vi "Module Loop.vi"(8 "error in (no error)":errorcluster, 11 "PluginGUI in":refnum<class "PluginGUI.lvclass">) -> (0 "error out":errorcluster, 3 "PluginGUI out":refnum<class "PluginGUI.lvclass">)   [LabVIEW 2020, in "VolatusGUI.lvlib" / "PluginGUI.lvclass"]
uses:
  PluginGUI.lvclass
  C:/dev/lv20CE/relink/lv-volatus/Volatus/Module/Module.lvclass
  Volatus/Module/Module.lvclass
  PluginGUI.lvclass/PluginGUI.ctl
  GUI Info.ctl
  Volatus/Show GUI Options.ctl
  Volatus/Module/Module.lvclass/Module.ctl
  <vilib>/Utility/error.llb/Error Cluster From Error Code.vi
  GUI Helper/GUI Helper.lvclass
  Volatus/Volatus.lvlib
  VolatusGUI.lvlib
  C:/dev/lv20CE/relink/lv-volatus/VolatusGUI/PluginGUI/PluginGUI.lvclass
  Volatus/Roles API/Roles API.lvclass
panel:
  out "VI Name":string
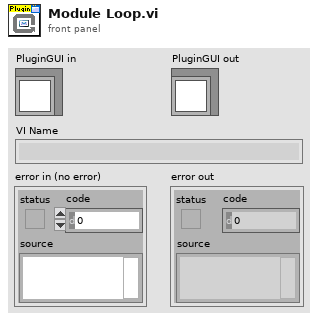
[diagram p1: front panel]
types:
  T1 = typedef "VolatusGUI.lvlib/GUI Info.ctl" = cluster{"Color":u32, "Name":string}
  T2 = typedef "Volatus.lvlib/Show GUI Options.ctl" = cluster{"Show Core Module":bool}
  T3 = enum32{"Invalid", "Standard", "Closed", "Hidden", "Minimized", "Maximized"}
  T4 = typedef "VolatusGUI.lvlib/PluginGUI.lvclass/GUI Type.ctl" = enum16{"Unknown", "Config", "Path", "Ref"}
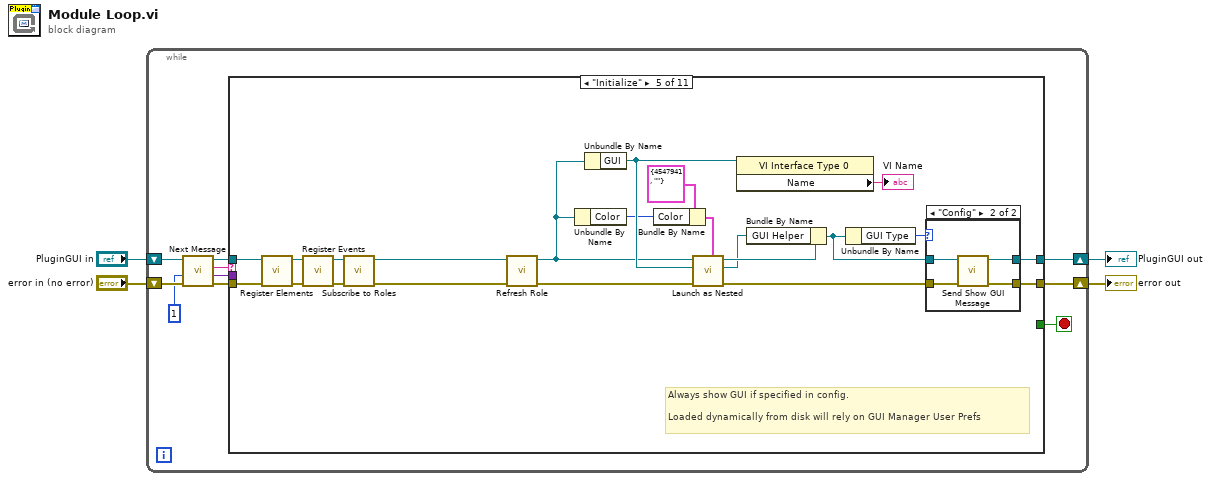
[diagram p0: block diagram]
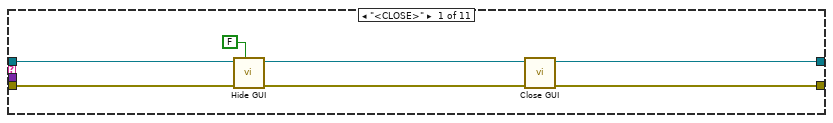
[diagram p2: hidden frame]
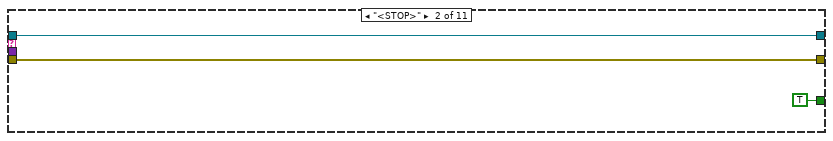
[diagram p3: hidden frame]
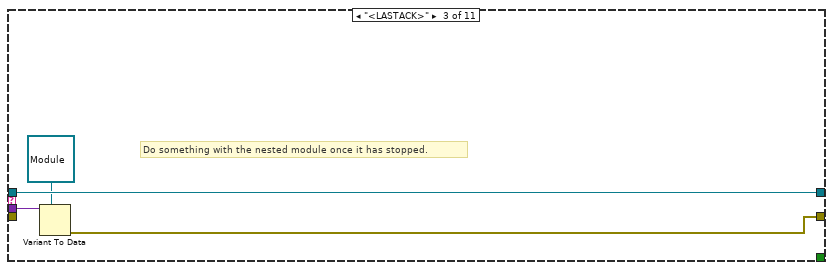
[diagram p4: hidden frame]
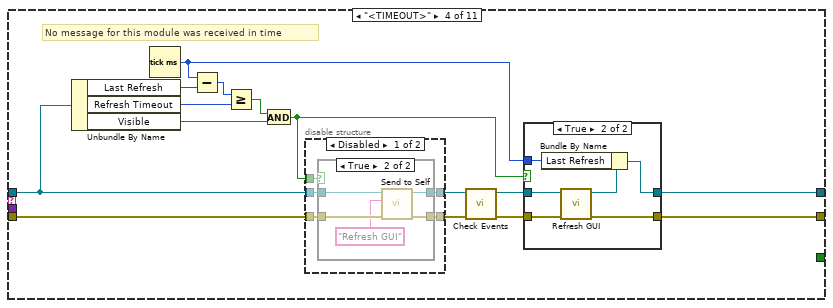
[diagram p5: hidden frame]
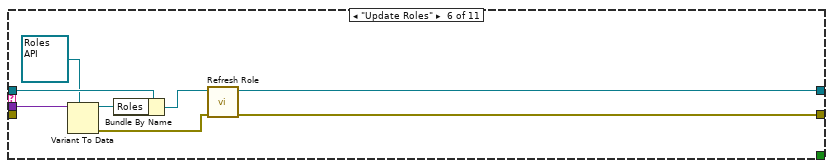
[diagram p10: hidden frame]
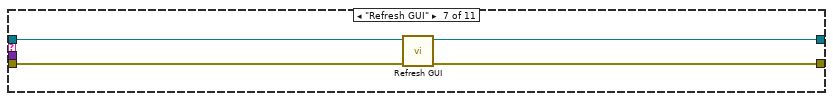
[diagram p11: hidden frame]
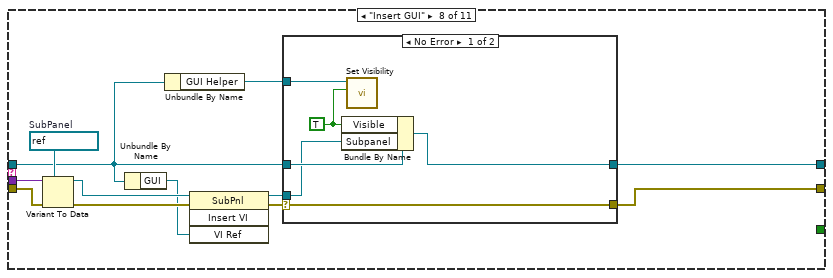
[diagram p12: hidden frame]
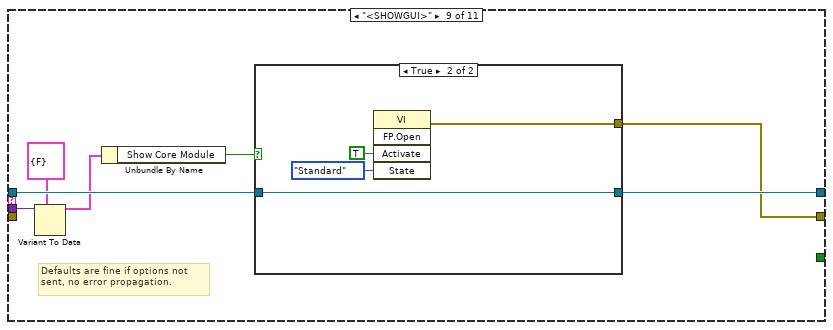
[diagram p14: hidden frame]
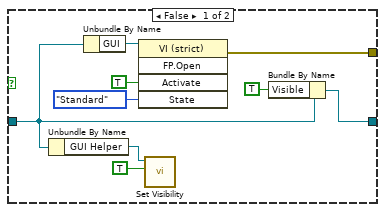
[diagram p15: hidden frame]
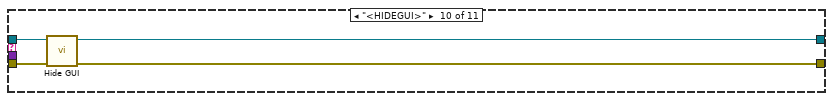
[diagram p16: hidden frame]
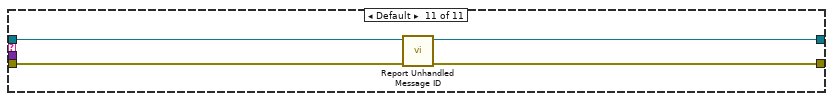
[diagram p17: hidden frame]
diagram:
  n1 = while {
    shift-right: [w9] -> w3
    shift-left: "PluginGUI in" -> [w14]
    shift-right: [w8] -> w2
    shift-left: "error in (no error)" -> [w13]
    stop <- w7 stop-if-true
    n2 = call "Next Message.vi"("error in (no error)"=w13, "Timeout ms (-1)"=1, "Module in"=w14) -> ("error out"=w12:errorcluster, "Data"=w6:variant, "ID"=w11:string, "Module in"=w10:refnum<class "PluginGUI.lvclass">)  [unwired: 5 in]
    n3 = case shown="\"Initialize\"" w11 {
      tunnel: w12 -> [w21 w23 _ w43 w84 _ w105 w117 _ w148 w153]
      tunnel: w10 -> [w19 w24 w28 w41 w74 w101 w103 w107 w131 w149 w151]
      tunnel: [w15 w24 w28 w31 w77 w96 w102 w109 w132 w147 w150] -> w9
      tunnel: [w17 w23 w25 w33 w78 w94 w104 w108 w126 w146 w152] -> w8
      tunnel: [_ TRUE _ _ _ _ _ _ _ _ _] -> w7
      tunnel: w6 -> [_ _ w27 _ _ w100 _ w116 w130 _ _]
      frame "<CLOSE>" {
        n4 = call "Hide GUI.vi"("Save Pref (T)"=FALSE, "error in (no error)"=w21, "PluginGUI in"=w19) -> ("error out"=w20:errorcluster, "PluginGUI out"=w16:refnum<class "PluginGUI.lvclass">)  [unwired: 7 in]
        n5 = call "Close GUI.vi"("error in (no error)"=w20, "PluginGUI in"=w16) -> ("error out"=w17:errorcluster, "PluginGUI out"=w15:refnum<class "PluginGUI.lvclass">)  [unwired: 8 in]
      }
      frame "<STOP>" {
      }
      frame "<LASTACK>" {
        # "Do something with the nested module once it has stopped."
        n6 = Variant To Data(type=refnum<class "Module.lvclass"> refnum ("Volatus:Module"), Variant=w27) -> (error out=w25:errorcluster)  [unwired: 1 in, 1 out]
      }
      frame "<TIMEOUT>" {
        # "No message for this module was received in time"
        n7 = Unbundle By Name(w41) -> ("Last Refresh"=w37:u32, "Refresh Timeout"=w36:i32, "Visible"=w40:bool)
        n8 = Tick Count (ms)() -> (millisecond timer value=w29:u32)
        n9 = Subtract(x=w29, y=w37) -> (x-y=w35:u32)
        n10 = Greater Or Equal?(x=w35, y=w36) -> (x >= y?=w34:bool)
        n11 = And(x=w34, y=w40) -> (x .and. y?=w30:bool)
        n12 = disable-structure shown="Disabled" {
          disable-tunnel: w43 -> [w56 w64]
          disable-tunnel: [w55 w64] -> w42
          disable-tunnel: w41 -> [w54 w65]
          disable-tunnel: [w53 w65] -> w38
          disable-tunnel: w30 -> [w52 _]
          frame Disabled {
            n13 = case shown="True" w52 {
              tunnel: w56 -> [w57 w63]
              tunnel: [w57 w62] -> w55
              tunnel: [w58 w61] -> w53
              tunnel: w54 -> [w58 w59]
              frame False {
              }
              frame True {
                n14 = call "Send to Self.vi"("error in (no error)"=w63, "Message ID"="Refresh GUI", "Module in"=w59) -> ("error out"=w62:errorcluster, "Module in"=w61:refnum<class "PluginGUI.lvclass">)  [unwired: 7 in]
              }
            }
          }
          frame Enabled {
          }
        }
        n15 = call "Check Events.vi"("error in (no error)"=w42, "PluginGUI in"=w38) -> ("error out"=w39:errorcluster, "PluginGUI out"=w32:refnum<class "PluginGUI.lvclass">)  [unwired: 8 in]
        n16 = case shown="True" w30 {
          tunnel: w39 -> [w44 w51]
          tunnel: [w44 w50] -> w33
          tunnel: w32 -> [w45 w49]
          tunnel: [w45 w47] -> w31
          tunnel: w29 -> [_ w46]
          frame False {
          }
          frame True {
            n17 = call "Refresh GUI.vi"("error in (no error)"=w51, "PluginGUI in"=w49) -> ("error out"=w50:errorcluster, "PluginGUI out"=w48:refnum<class "PluginGUI.lvclass">)  [unwired: 8 in]
            n18 = Bundle By Name(cluster=w48, "Last Refresh"=w46) -> (w47:refnum<class "PluginGUI.lvclass">)
          }
        }
      }
      frame "Initialize" {
        # "Always show GUI if specified in config.\n\nLoaded dynamically from disk will rely on GUI Manager User Prefs"
        n19 = call "Register Elements.vi"("error in (no error)"=w84, "PluginGUI in"=w74) -> ("error out"=w87:errorcluster, "PluginGUI out"=w85:refnum<class "PluginGUI.lvclass">)  [unwired: 8 in]
        n20 = call "Register Events.vi"("error in (no error)"=w87, "PluginGUI in"=w85) -> ("error out"=w86:errorcluster, "PluginGUI out"=w69:refnum<class "PluginGUI.lvclass">)  [unwired: 8 in]
        n21 = call "Subscribe to Roles.vi"("error in (no error)"=w86, "Module in"=w69) -> ("error out"=w70:errorcluster, "Module out"=w67:refnum<class "PluginGUI.lvclass">)  [unwired: 8 in]
        n22 = call "Refresh Role.vi"("error in (no error)"=w70, "PluginGUI in"=w67) -> ("error out"=w68:errorcluster, "PluginGUI out"=w66:refnum<class "PluginGUI.lvclass">)  [unwired: 8 in]
        n23 = Unbundle By Name(w66) -> ("Color"=w71:u32)
        n24 = Unbundle By Name(w66) -> ("GUI"=w80:refnum<vi>)
        n25 = Bundle By Name(cluster=T1 {"Color"=4547941, "Name"=""} ("GUI Info (Default)"), "Color"=w71) -> (w72:T1)
        n26 = call "Launch as Nested.vi"("GUI Info (Default)"=w72, "error in (no error)"=w68, "GUI"=w80, "Parent in"=w66) -> ("error out"=w82:errorcluster, "MessageQ"=w79:refnum<class "MessageQ.lvclass">, "Parent"=w81:refnum<class "PluginGUI.lvclass">)  [unwired: 5 in]
        n27 = property class="VI Interface Type 0"(reference=w80) -> ("Name"=→"VI Name":string)  [unwired: 1 in, 2 out]
        n28 = Bundle By Name(cluster=w81, "GUI Helper"=w79) -> (w76:refnum<class "PluginGUI.lvclass">)
        n29 = Unbundle By Name(w76) -> ("GUI Type"=w75:T4)
        n30 = case shown="\"Config\"" w75 {
          tunnel: w82 -> [w88 w93]
          tunnel: [w88 w92] -> w78
          tunnel: [w89 w91] -> w77
          tunnel: w76 -> [w89 w90]
          frame Default {
          }
          frame "Config" {
            n31 = call "Send Show GUI Message.vi"("error in (no error)"=w93, "Module in"=w90) -> ("error out"=w92:errorcluster, "Module in"=w91:refnum<class "PluginGUI.lvclass">)  [unwired: 8 in]
          }
        }
      }
      frame "Update Roles" {
        n32 = Variant To Data(type=refnum<class "Roles API.lvclass"> refnum ("Volatus:Roles API.lvclass"), Variant=w100) -> (data=w97:refnum<class "Roles API.lvclass">, error out=w95:errorcluster)  [unwired: 1 in]
        n33 = Bundle By Name(cluster=w101, "Roles"=w97) -> (w98:refnum<class "PluginGUI.lvclass">)
        n34 = call "Refresh Role.vi"("error in (no error)"=w95, "PluginGUI in"=w98) -> ("error out"=w94:errorcluster, "PluginGUI out"=w96:refnum<class "PluginGUI.lvclass">)  [unwired: 8 in]
      }
      frame "Refresh GUI" {
        n35 = call "Refresh GUI.vi"("error in (no error)"=w105, "PluginGUI in"=w103) -> ("error out"=w104:errorcluster, "PluginGUI out"=w102:refnum<class "PluginGUI.lvclass">)  [unwired: 8 in]
      }
      frame "Insert GUI" {
        w115 = refnum<vi> refnum  # SubPanel
        n36 = Variant To Data(error in=w117, type=w115, Variant=w116) -> (data=w113:refnum<vi>, error out=w114:errorcluster)
        n37 = Unbundle By Name(w107) -> ("GUI"=w112:refnum<vi>)
        n38 = Unbundle By Name(w107) -> ("GUI Helper"=w106:refnum<class "MessageQ.lvclass">)
        n39 = invoke class="SubPnl" method="Insert VI"(reference=w113, error in=w114, "VI Ref"=w112) -> (reference out=w110:refnum<vi>, error out=w111:errorcluster)  [unwired: 1 in, 2 out]
        n40 = case shown="No Error" w111 {
          selector: w111 -> [w120 w125]
          tunnel: w107 -> [w123 w124]
          tunnel: w110 -> [w122 _]
          tunnel: [w121 w124] -> w109
          tunnel: [w120 w125] -> w108
          tunnel: w106 -> [w119 _]
          frame No Error {
            w118 = TRUE ("Visible")
            n41 = Bundle By Name(cluster=w123, "Visible"=w118, "Subpanel"=w122) -> (w121:refnum<class "PluginGUI.lvclass">)
            n42 = call "Set Visibility.vi"("Visible"=w118, "GUI Helper in"=w119) -> ()  [unwired: 8 in, 2 out]
          }
          frame Error {
          }
        }
      }
      frame "<SHOWGUI>" {
        # "Defaults are fine if options not sent, no error propagation."
        n43 = Variant To Data(type=T2 {"Show Core Module"=FALSE} ("Show GUI Options"), Variant=w130) -> (data=w128:T2)  [unwired: 1 in, 1 out]
        n44 = Unbundle By Name(w128) -> ("Show Core Module"=w127:bool)
        n45 = case shown="True" w127 {
          tunnel: [w138 w145] -> w132
          tunnel: w131 -> [w136 w145]
          tunnel: [w133 w142] -> w126
          frame False {
            n46 = Unbundle By Name(w136) -> ("GUI Helper"=w135:refnum<class "MessageQ.lvclass">)
            n47 = Unbundle By Name(w136) -> ("GUI"=w141:refnum<vi>)
            n48 = invoke class="VI (strict)" method="FP.Open"(reference=w141, "Activate"=TRUE ("Activate?"), "State"=T3."Standard") -> (error out=w133:errorcluster)  [unwired: 2 in, 4 out]
            n49 = call "Set Visibility.vi"("Visible"=TRUE, "GUI Helper in"=w135) -> ()  [unwired: 8 in, 2 out]
            n50 = Bundle By Name(cluster=w136, "Visible"=TRUE) -> (w138:refnum<class "PluginGUI.lvclass">)
          }
          frame True {
            n51 = invoke class="VI" method="FP.Open"("Activate"=TRUE ("Activate?"), "State"=T3."Standard") -> (error out=w142:errorcluster)  [unwired: 3 in, 4 out]
          }
        }
      }
      frame "<HIDEGUI>" {
        n52 = call "Hide GUI.vi"("error in (no error)"=w148, "PluginGUI in"=w149) -> ("error out"=w146:errorcluster, "PluginGUI out"=w147:refnum<class "PluginGUI.lvclass">)  [unwired: 8 in]
      }
      frame Default {
        n53 = call "Report Unhandled Message ID.vi"("error in (no error)"=w153, "Module in"=w151) -> ("error out"=w152:errorcluster, "Module in"=w150:refnum<class "PluginGUI.lvclass">)  [unwired: 8 in]
      }
    }
  }
  "error out" <- w2
  "PluginGUI out" <- w3
